vi "Read Index of Plugin.vi"(8 "error in (no error)":errorcluster, 11 "Plugin Handler Launch Plugin in":refnum<class "Plugin Handler Launch Plugin.lvclass">) -> (0 "error out":errorcluster, 2 "Index of Plugin":i32, 3 "Plugin Handler Launch Plugin out":refnum<class "Plugin Handler Launch Plugin.lvclass">)   [LabVIEW 2011, in "Plugin Handler Launch Plugin.lvclass"]
uses:
  Plugin Handler Launch Plugin.lvclass
  Plugin Handler Launch Plugin.lvclass/Plugin Handler Launch Plugin.ctl
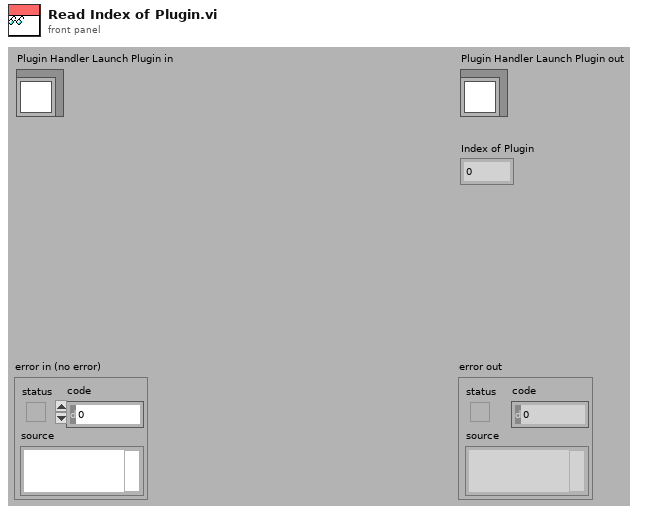
[diagram p1: front panel]
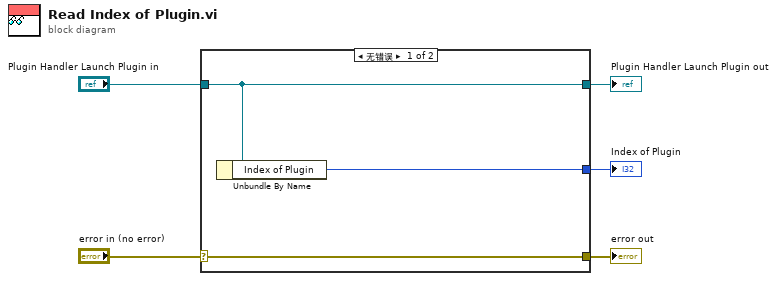
[diagram p0: block diagram]
diagram:
  n1 = case shown="无错误" "error in (no error)" {
    selector: "error in (no error)" -> [w8 w9]
    tunnel: [w8 w9] -> w4
    tunnel: [w7 w10] -> w2
    tunnel: "Plugin Handler Launch Plugin in" -> [w7 w10]
    tunnel: [w6 _] -> w1
    frame No Error {
      n2 = Unbundle By Name(w7) -> ("Index of Plugin"=w6:i32)
    }
    frame Error {
    }
  }
  "error out" <- w4
  "Plugin Handler Launch Plugin out" <- w2
  "Index of Plugin" <- w1
